vi "AddTiffPage_I16_text_res.vi"(0 "TIFF file":T2 {"BigTiff,Endian" items=["Big-Endian"=0, "Native"=1, "Little-Endian"=2, "BigTiff-Big-Endian"=256, "Bigtiff,Native"=257, "Biftiff,Littleendian"=258]}, 1 "After last DIROffset":u64=8 format="%.0x", 2 "Text":string="test", 3 "16-bit pixmap x, y":i16[][](array[numeric]), 4 "Pixelsize [µm]":T1={"Xpixelsize[µm]"=1e-06, "Ypixelsize[µm]"=1e-06}) -> (5 "TIFF file":T2 {"BigTiff,Endian" items=["Big-Endian"=0, "Native"=1, "Little-Endian"=2, "BigTiff-Big-Endian"=256, "Bigtiff,Native"=257, "Biftiff,Littleendian"=258]}, 6 "AfterDIRoffset":u64 format="%.0x", 7 "error out":errorcluster)   [LabVIEW 2011]
panel:
  out "IFD-Offste written":i64 format="%.0x"
  in  "error in":errorcluster
  out "eof\nstart here":i64
  out "size(s)":i32[](array[numeric])
  out "Directory Entries":T3(array[cluster])
  # "the 4/8 bytes before will be changed"
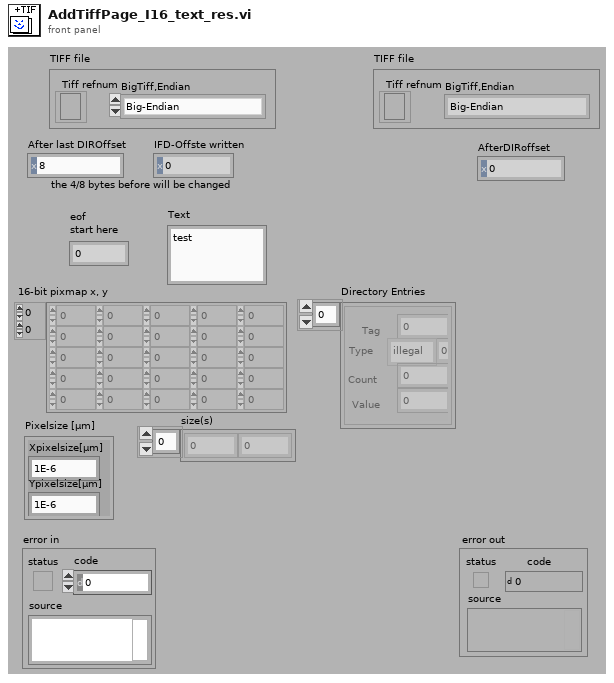
[diagram p1: front panel]
types:
  T1 = cluster{"Xpixelsize[µm]":sgl, "Ypixelsize[µm]":sgl}
  T2 = cluster{"Tiff refnum":refnum<file>, "BigTiff,Endian":u16}
  T3 = cluster{"Tag":u16, "Type":enum16{"illegal", "Byte", "Ascii", "Short", "Long"}, "Count":u32, "Value":u32}[]
  T4 = cluster{"offset (in bytes)":i64, "offset (in bytes)":i64}
  T5 = typedef "IFD.ctl" = cluster{"Tag":u16, "Type":enum16{"illegal", "Byte", "Ascii", "Short", "Long", "Rational", "SByte", "Undefined", "SShort", "SLong", "SRational 2xSLong", "Float 4byte", "Double 8Byte", "No13", "No14", "No15", "U64", "I64", "U64-IFD8"}, "Count":u64, "Value":u64}
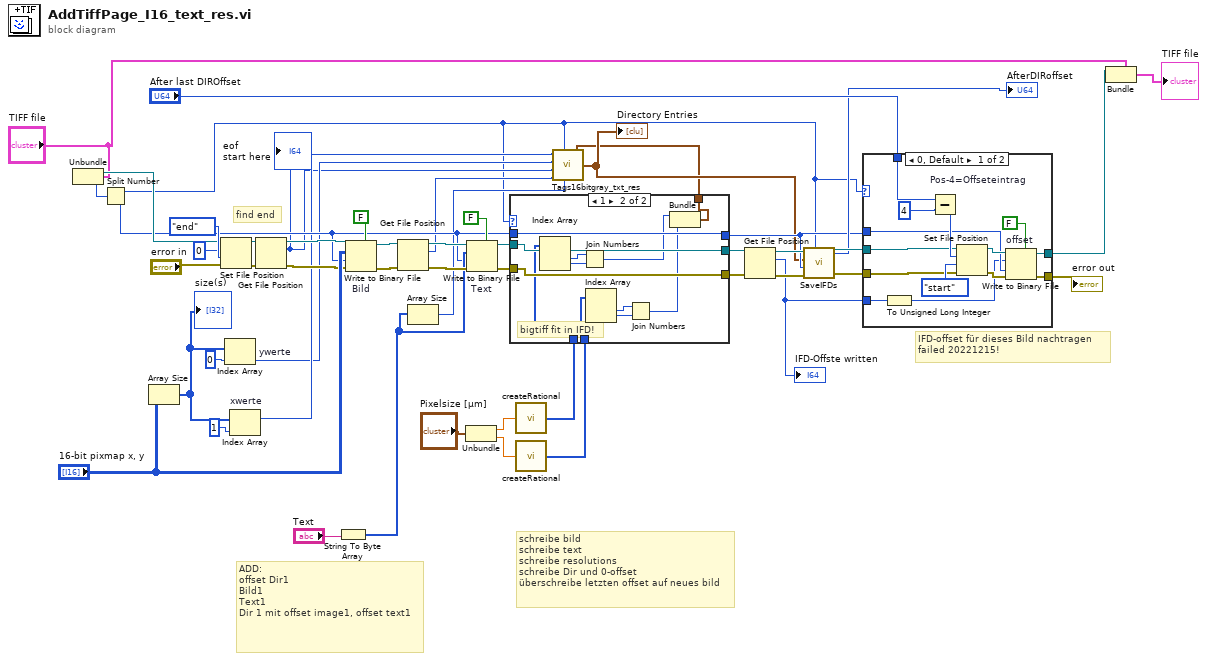
[diagram p0: block diagram]
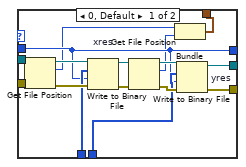
[diagram p2: hidden frame]
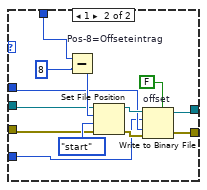
[diagram p3: hidden frame]
diagram:
  # "IFD-offset für dieses Bild nachtragen\nfailed 20221215!"
  # "find end"
  # "schreibe bild\nschreibe text\nschreibe resolutions\nschreibe Dir und 0-offset\nüberschreibe letzten offset auf neues bild"
  # "ADD:\noffset Dir1\nBild1\nText1\nDir 1 mit offset image1, offset text1"
  n1 = Unbundle("TIFF file") -> ("Tiff refnum"=w36:refnum<file>, "BigTiff,Endian"=w26:u16)
  n2 = Split Number(x=w26) -> (hi(x)=w3:u8, lo(x)=w10:u8)
  n3 = Array Size(array="16-bit pixmap x, y") -> (size(s)=w49:i32[])
  "size(s)" <- w49
  n4 = Set File Position(offset (in bytes) (0)=0 ("pos offset (0)"), refnum=w36, from (0:start)=enum16{"start", "end", "current"}."end" ("pos mode (0:2)"), error in="error in") -> (refnum out=w42:refnum<file>, error out=w41:errorcluster)
  n5 = Index Array "ywerte"(array=w49, index=0 ("Index")) -> (element=w7:i32)
  n6 = Index Array "xwerte"(array=w49, index=1 ("Index")) -> (element=w8:i32)
  n7 = Get File Position(4:w41, 7:w42) -> (0:w34:errorcluster, 2:w6:i64, 3:w35:refnum<file>)
  "eof\nstart here" <- w6
  n8 = String To Byte Array(string="Text") -> (unsigned byte array=w27:u8[])
  n9 = Write to Binary File "Bild"(file (use dialog)=w35, data="16-bit pixmap x, y", error in=w34, 5:FALSE ("Array- oder Stringgröße voranstellen? (T)"), 9:w10) -> (refnum out=w39:refnum<file>, error out=w38:errorcluster)  [unwired: 2 out]
  n10 = Get File Position(4:w38, 7:w39) -> (0:w33:errorcluster, 2:w5:i64, 3:w32:refnum<file>)
  n11 = Array Size(array=w27) -> (size(s)=w4:i32)
  n12 = Unbundle("Pixelsize [µm]") -> ("Xpixelsize[µm]"=w18:sgl, "Ypixelsize[µm]"=w19:sgl)
  n13 = Write to Binary File "Text"(file (use dialog)=w32, data=w27, error in=w33, 5:FALSE ("Array- oder Stringgröße voranstellen? (T)"), 9:w10) -> (refnum out=w14:refnum<file>, error out=w16:errorcluster)  [unwired: 2 out]
  n14 = call "createRational.vi"("real"=w18) -> ("rational 2xU32"=w12:u32[])
  n15 = call "createRational.vi"("real"=w19) -> ("rational 2xU32"=w11:u32[])
  n16 = case shown="1" w3 {
    tunnel: w16 -> [w65 w77]
    tunnel: [w62 w77] -> w15
    tunnel: w14 -> [w61 w78]
    tunnel: [w58 w78] -> w13
    tunnel: w12 -> [w57 w76]
    tunnel: w11 -> [w56 w71]
    tunnel: w10 -> [w55 w79]
    tunnel: [w55 w79] -> w9
    tunnel: [w52 w68] -> w1
    frame 0, Default {
      n17 = Get File Position(4:w65, 7:w61) -> (0:w64:errorcluster, 2:w54:i64, 3:w60:refnum<file>)
      n18 = Write to Binary File "xres"(file (use dialog)=w60, data=w57, error in=w64, 9:w55) -> (refnum out=w67:refnum<file>, error out=w66:errorcluster)  [unwired: 1 in, 2 out]
      n19 = Get File Position(4:w66, 7:w67) -> (0:w63:errorcluster, 2:w53:i64, 3:w59:refnum<file>)
      n20 = Bundle("offset (in bytes)"=w54, "offset (in bytes)"=w53) -> (w52:T4)  [unwired: 1 in]
      n21 = Write to Binary File "yres"(file (use dialog)=w59, data=w56, error in=w63, 9:w55) -> (refnum out=w58:refnum<file>, error out=w62:errorcluster)  [unwired: 1 in, 2 out]
    }
    frame 1 {
      # "bigtiff fit in IFD!"
      n22 = Index Array(array=w76) -> (element #1=w75:u32, element #2=w74:u32)  [unwired: 2 in]
      n23 = Join Numbers(hi=w75, lo=w74) -> ((hi.lo)=w70:u64)
      n24 = Index Array(array=w71) -> (element #1=w73:u32, element #2=w72:u32)  [unwired: 2 in]
      n25 = Join Numbers(hi=w73, lo=w72) -> ((hi.lo)=w69:u64)
      n26 = Bundle(w70, w69) -> (w68:cluster{u64, u64})  [unwired: 1 in]
    }
  }
  n27 = call "Tags16bitgray_txt_res.vi"("xbreite"=w8, "BigTiff"=w3, "yhöhe"=w7, "BildOffset Bytes"=w6, "Text length"=w4, "Text Offset Bytes"=w5, "Cluster"=w1) -> ("Directory Entrys"=w2:T5[])  [unwired: 1 in]
  "Directory Entries" <- w2
  n28 = Get File Position(4:w15, 7:w13) -> (0:w25:errorcluster, 2:w20:i64, 3:w24:refnum<file>)
  "IFD-Offste written" <- w20
  n29 = call "SaveIFDs.vi"("BigTiff"=w3, "Fehler (Eingang)"=w25, "Byte-Reihenfolge (0:Big-Endian, Netzwerkreihenfolge)"=w9, "IFDs"=w2, "Refnum"=w24) -> ("Fehler (Ausgang)"=w22:errorcluster, "after next offset (zero)"=→"AfterDIRoffset":i64, "Refnum (Ausgang)"=w23:refnum<file>)  [unwired: 4 out]
  n30 = case shown="0, Default" w3 {
    tunnel: "After last DIROffset" -> [w90 w94]
    tunnel: [w89 w95] -> w43
    tunnel: [w85 w96] -> w31
    tunnel: w9 -> [w84 w100]
    tunnel: w23 -> [w83 w99]
    tunnel: w22 -> [w82 w98]
    tunnel: w20 -> [w81 w97]
    frame 0, Default {
      n31 = To Unsigned Long Integer(number=w81) -> (unsigned 32bit integer=w80:u32)
      n32 = Subtract "Pos-4=Offseteintrag"(x=w90, y=u32 4) -> (x-y=w91:u64)
      n33 = Set File Position(offset (in bytes) (0)=w91, refnum=w83, from (0:start)=enum16{"start", "end", "current"}."start" ("pos mode (0:2)"), error in=w82) -> (refnum out=w88:refnum<file>, error out=w87:errorcluster)
      n34 = Write to Binary File "offset"(file (use dialog)=w88, data=w80, error in=w87, 5:FALSE ("Array- oder Stringgröße voranstellen? (T)"), 9:w84) -> (refnum out=w85:refnum<file>, error out=w89:errorcluster)  [unwired: 2 out]
    }
    frame 1 {
      n35 = Subtract "Pos-8=Offseteintrag"(x=w94, y=u32 8) -> (x-y=w104:u64)
      n36 = Set File Position(offset (in bytes) (0)=w104, refnum=w99, from (0:start)=enum16{"start", "end", "current"}."start" ("pos mode (0:2)"), error in=w98) -> (refnum out=w103:refnum<file>, error out=w102:errorcluster)
      n37 = Write to Binary File "offset"(file (use dialog)=w103, data=w97, error in=w102, 5:FALSE ("Array- oder Stringgröße voranstellen? (T)"), 9:w100) -> (refnum out=w96:refnum<file>, error out=w95:errorcluster)  [unwired: 2 out]
    }
  }
  "error out" <- w43
  n38 = Bundle(cluster="TIFF file", "Tiff refnum"=w31) -> (→"TIFF file":T2)  [unwired: 1 out]
